vi "From Variant.vi"(8 "Error In":errorcluster, 10 "Variant":variant, 11 "2D Flt In":refnum<class "2D Flt.lvclass">) -> (0 "Error Out":errorcluster, 3 "2D Flt Out":refnum<class "2D Flt.lvclass">)   [LabVIEW 2017, in "Tree API.lvlib" / "2D Flt.lvclass"]
doc: "Dynamic dispatch interface for conversion of variant LV data to Tree Data classes."
uses:
  2D Flt.lvclass
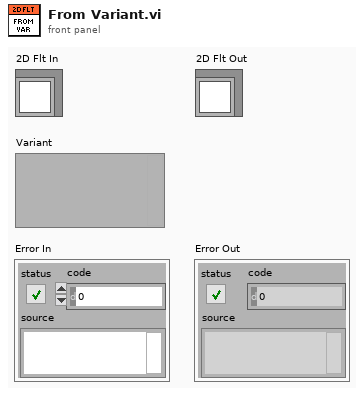
[diagram p1: front panel]
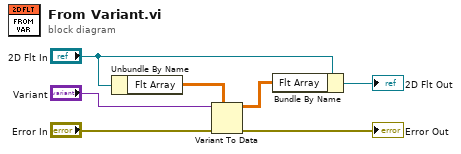
[diagram p0: block diagram]
diagram:
  n1 = Unbundle By Name("2D Flt In") -> ("Flt Array"=w5:dbl[][])
  n2 = Variant To Data(error in="Error In", type=w5, Variant="Variant") -> (data=w3:dbl[][], error out=→"Error Out":errorcluster)
  n3 = Bundle By Name(cluster="2D Flt In", "Flt Array"=w3) -> (→"2D Flt Out":refnum<class "2D Flt.lvclass">)
